vi "Post-Init.vi"(8 "error in (no error)":errorcluster, 11 "Pulse Driver in":refnum<class "Pulse Driver.lvclass">) -> (0 "error out":errorcluster, 2 "Init Result":refnum<class "Acquired Result.lvclass">, 3 "Pulse Driver out":refnum<class "Pulse Driver.lvclass">)   [LabVIEW 2016, in "Pulse Driver.lvclass"]
uses:
  Pulse Driver.lvclass
  C:/github/NHMFL_Core/Libraries/Instruments/Instrument Driver/Instrument Driver.lvclass
  Measure_core/Results/Acquired Result/Acquired Result.lvclass
  Instrument Driver/Instrument Driver.lvclass/Instrument Driver.ctl
  Pulse Driver.lvclass/Pulse Driver.ctl
  Measure_core/Results/Acquired Result/Acquired Result.lvclass/Acquired Result.ctl
  Instrument Driver/Read Channel names.vi
  Write Current read position.vi
  Instrument Driver/Write Channel names.vi
  Write t0.vi
  Write dt.vi
  Measure_core/Results/Acquired Result/Write Channels.vi
  Read Pulse Configuration.vi
  Instrument Driver/Instrument Driver.lvclass
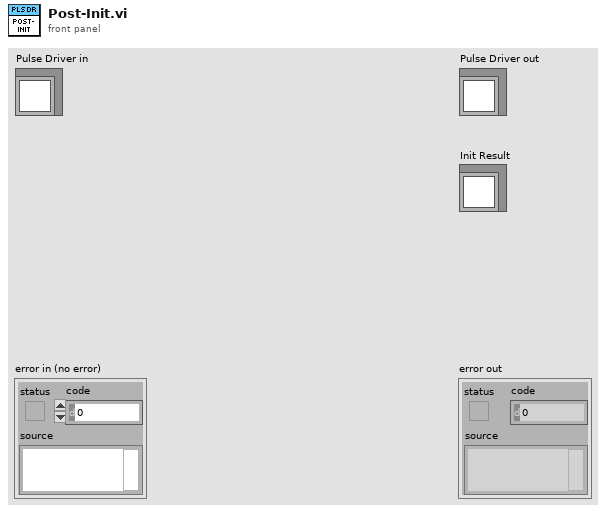
[diagram p1: front panel]
types:
  T1 = typedef "Pusle Driver Configuration.ctl" = cluster{"Pre-trigger duration":dbl, "Post-trigger duration":dbl, "Rate":dbl, "Ranges":dbl[], "Re-name channels":string[], "Active channels":string, "External clock":bool}
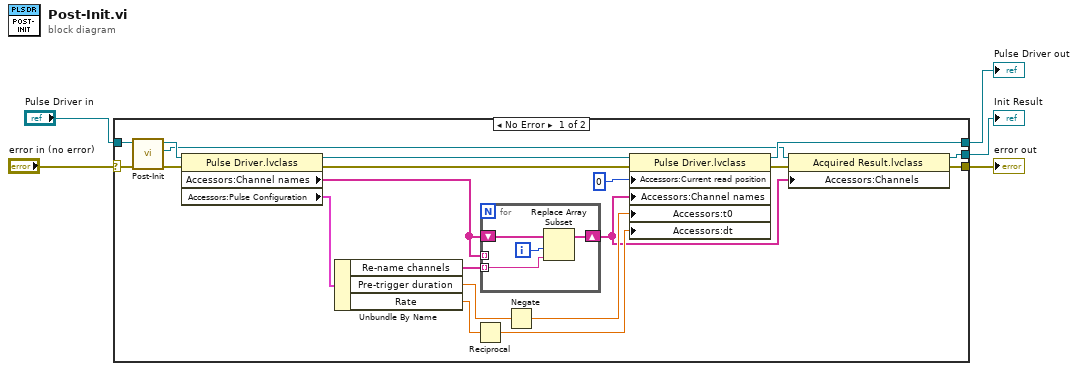
[diagram p0: block diagram]
diagram:
  n1 = case shown="No Error" "error in (no error)" {
    selector: "error in (no error)" -> [w7 w31]
    tunnel: [w12 w31] -> w4
    tunnel: [w24 w30] -> w2
    tunnel: "Pulse Driver in" -> [w22 w30]
    tunnel: [w10 _] -> w1
    frame No Error {
      n2 = call-parent "Post-Init.vi"("error in (no error)"=w7, "Instrument Driver in"=w22) -> ("error out"=w6:errorcluster, "Init Result"=w8:refnum<class "Acquired Result.lvclass">, "Instrument Driver out"=w9:refnum<class "Pulse Driver.lvclass">)  [unwired: 7 in]
      n3 = property class="Pulse Driver.lvclass"(reference=w9, error in=w6) -> (reference out=w17:refnum<class "Pulse Driver.lvclass">, error out=w18:errorcluster, "Accessors:Channel names"=w19:string[], "Accessors:Pulse Configuration"=w21:T1)
      n4 = Unbundle By Name(w21) -> ("Re-name channels"=w20:string[], "Pre-trigger duration"=w16:dbl, "Rate"=w14:dbl)
      n5 = Reciprocal(x=w14) -> (1/x=w13:dbl)
      n6 = for {
        tunnel: w20 -> [w27] mode=indexing
        shift-right: [w26] -> w11
        shift-left: w19 -> [w29]
        tunnel: w19 -> [_] mode=indexing
        i -> [w28]
        n7 = Replace Array Subset(array=w29, new element=w27, index=w28) -> (w26:string[])
      }
      n8 = Negate(x=w16) -> (-x=w15:dbl)
      n9 = property class="Pulse Driver.lvclass"(reference=w17, error in=w18, "Accessors:Current read position"=0 ("Current read position"), "Accessors:Channel names"=w11, "Accessors:t0"=w15, "Accessors:dt"=w13) -> (reference out=w24:refnum<class "Pulse Driver.lvclass">, error out=w23:errorcluster)
      n10 = property class="Acquired Result.lvclass"(reference=w8, error in=w23, "Accessors:Channels"=w11) -> (reference out=w10:refnum<class "Acquired Result.lvclass">, error out=w12:errorcluster)
    }
    frame Error {
    }
  }
  "error out" <- w4
  "Pulse Driver out" <- w2
  "Init Result" <- w1
